vi "Split.vi"(6 "Groups":string[][](array[string]), 8 "error in (no error)":errorcluster caption="entrée d'erreur (pas d'erreur)", 9 "y":string[][](array[string]), 10 "X":string[][](array[string]), 11 "StratifiedKFold.lvclass":refnum<class "StratifiedKFold.lvclass">) -> (0 "error out":errorcluster caption="sortie d'erreur", 2 "Split":T1(array[cluster]), 3 "StratifiedKFold.lvclass":refnum<class "StratifiedKFold.lvclass">)   [LabVIEW 2020, in "StratifiedKFold.lvclass"]
doc: "Returns : \n\n- train : ndarray\n The training set indices for that split.\n\n- test : ndarray\n The testing set indices for that split."
uses:
  StratifiedKFold.lvclass
  StratifiedKFold.lvclass/StratifiedKFold.ctl
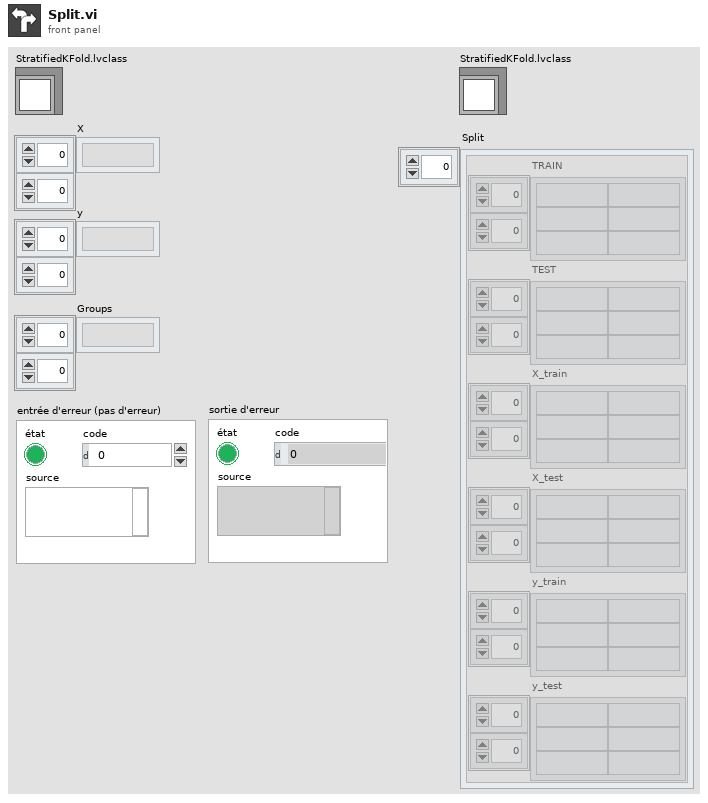
[diagram p1: front panel]
types:
  T1 = cluster{"TRAIN":string[][], "TEST":string[][], "X_train":string[][], "X_test":string[][], "y_train":string[][], "y_test":string[][]}[]
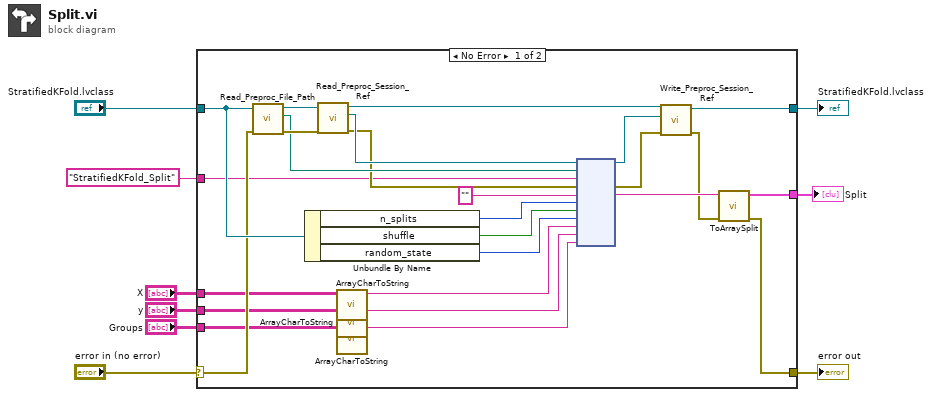
[diagram p0: block diagram]
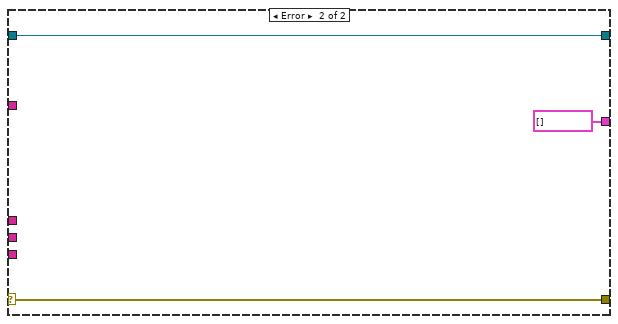
[diagram p2: hidden frame]
diagram:
  n1 = case shown="No Error" "error in (no error)" {
    selector: "error in (no error)" -> [w25 w38]
    tunnel: [w18 w38] -> w8
    tunnel: [w17 w37] -> w6
    tunnel: "StratifiedKFold.lvclass" -> [w26 w37]
    tunnel: "StratifiedKFold_Split" -> [w24 _]
    tunnel: "X" -> [w15 _]
    tunnel: "y" -> [w13 _]
    tunnel: "Groups" -> [w11 _]
    tunnel: [w16 T1 [] ("Split")] -> w1
    frame No Error {
      n2 = call-dynamic "Read_Preproc_File_Path.vi"("error in (no error)"=w25, "Python in"=w26) -> ("error out"=w34:errorcluster, "File_Path"=w33:path, "Python out"=w35:refnum<class "StratifiedKFold.lvclass">)  [unwired: 7 in]
      n3 = Unbundle By Name(w26) -> ("n_splits"=w23:i32, "shuffle"=w22:bool, "random_state"=w21:i32)
      n4 = call-dynamic "Read_Preproc_Session_Ref.vi"("error in (no error)"=w34, "Python in"=w35) -> ("error out"=w31:errorcluster, "Session_ref"=w32:refnum<k35>, "Python out"=w30:refnum<class "StratifiedKFold.lvclass">)  [unwired: 7 in]
      n5 = call "ArrayCharToString.vi"("TAB"=w15) -> ("Instruction"=w14:string)  [unwired: 10 in]
      n6 = call "ArrayCharToString.vi"("TAB"=w13) -> ("Instruction"=w12:string)  [unwired: 10 in]
      n7 = call "ArrayCharToString.vi"("TAB"=w11) -> ("Instruction"=w10:string)  [unwired: 10 in]
      n8 = node(w32, w33, w24, w31, "", w23, w22, w21, w14, w12, w10) -> (w28:refnum<k35>, w29:errorcluster, w20:string)  [unwired: 6 in, 2 out]
      n9 = call-dynamic "Write_Preproc_Session_Ref.vi"("error in (no error)"=w29, "Session_ref"=w28, "Python in"=w30) -> ("error out"=w19:errorcluster, "Python out"=w17:refnum<class "StratifiedKFold.lvclass">)  [unwired: 7 in]
      n10 = call "ToArraySplit.vi"("sortie d'erreur"=w19, "Return value"=w20) -> ("sortie d'erreur"=w18:errorcluster, "Split"=w16:T1)  [unwired: 8 in]
    }
    frame Error {
    }
  }
  "error out" <- w8
  "StratifiedKFold.lvclass" <- w6
  "Split" <- w1
